vi "Pathloss Folder Path.vi"() -> (2 "Pathloss Folder Path":path)   [LabVIEW 2012]
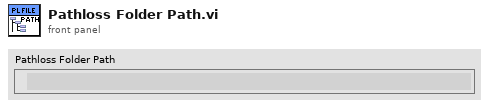
[diagram p1: front panel]
types:
  T1 = enum32{"invalid app kind", "Development System", "Run Time System", "Student Edition", "Embedded LabVIEW", "Evaluation", "Custom"}
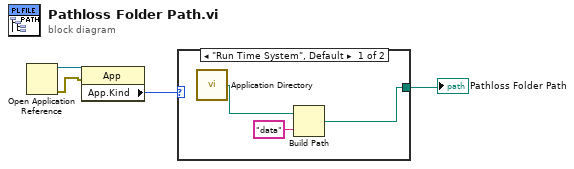
[diagram p0: block diagram]
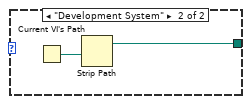
[diagram p2: hidden frame]
diagram:
  n1 = Open Application Reference() -> (0:w3:errorcluster, 3:w4:refnum<vi>)  [unwired: 4 in]
  n2 = property class="App"(reference=w4, error in=w3) -> ("App.Kind"=w2:T1)  [unwired: 2 out]
  n3 = case shown="\"Run Time System\", Default" w2 {
    tunnel: [w5 w8] -> w1
    frame "Run Time System", Default {
      n4 = call <vilib>:"Application Directory.vi"() -> ("Application Directory"=w7:path)
      n5 = Build Path(base path=w7, name or relative path="data") -> (appended path=w5:path)
    }
    frame "Development System" {
      n6 = Current VI's Path() -> (path=w9:path)
      n7 = Strip Path(path=w9) -> (stripped path=w8:path)  [unwired: 1 out]
    }
  }
  "Pathloss Folder Path" <- w1
